vi "LogHeader.vi"(11 "Data folder":path=path "C:/Data") -> (0 "error out":errorcluster, 3 "refnum out":refnum<file>)   [LabVIEW 2018]
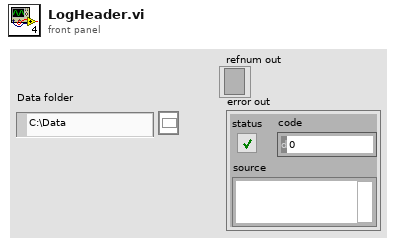
[diagram p1: front panel]
types:
  T1 = enum16{"open", "replace", "create", "open or create", "replace or create", "replace or create with confirmation"}
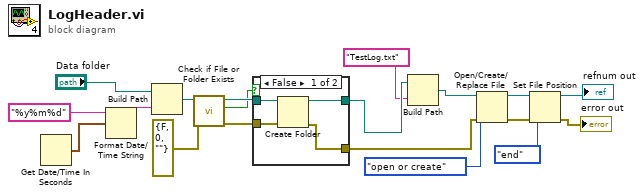
[diagram p0: block diagram]
diagram:
  n1 = Get Date/Time In Seconds() -> (seconds since 1Jan1904=w17:timestamp)
  n2 = Format Date/Time String(time format string (%c)="%y%m%d", seconds (now)=w17) -> (date/time string=w16:string)  [unwired: 1 in]
  n3 = Build Path(base path="Data folder", name or relative path=w16) -> (appended path=w15:path)
  n4 = call <vilib>:"Check if File or Folder Exists.vi"("error in (no error)"=errorcluster {"status"=FALSE, "code"=0, "source"=""}, "path"=w15) -> ("error out"=w11:errorcluster, "file or folder exists?"=w13:bool, "dup path"=w14:path)  [unwired: 7 in]
  n5 = case shown="False" w13 {
    tunnel: w14 -> [w23 w25]
    tunnel: [w22 w25] -> w12
    tunnel: w11 -> [w21 w24]
    tunnel: [w20 w24] -> w9
    frame False {
      n6 = Create Folder(path (use dialog)=w23, error in=w21) -> (created path=w22:path, error out=w20:errorcluster)  [unwired: 1 in, 1 out]
    }
    frame True {
    }
  }
  n7 = Build Path(base path=w12, name or relative path="TestLog.txt" ("input 2")) -> (appended path=w10:path)
  n8 = Open/Create/Replace File(file path (use dialog)=w10, error in=w9, operation (0:open)=T1."open or create") -> (refnum out=w3:refnum<file>, error out=w5:errorcluster)  [unwired: 3 in, 1 out]
  n9 = Set File Position(refnum=w3, from (0:start)=enum16{"start", "end", "current"}."end", error in=w5) -> (refnum out=→"refnum out":refnum<file>, error out=→"error out":errorcluster)  [unwired: 1 in]
